vi "Kv_correz_2024.vi"(2 "3rd ac pressure Virial \"G\" (Pa^-2)":dbl, 3 "Pressure [Pa]":dbl, 4 "2nd ac pressure Virial \"F\" (Pa^-1)":dbl) -> (1 "Kv":dbl)   [LabVIEW 2016]
uses:
  2022/SOS_Global_2022.vi
panel:
  out "Kv (ppm)":dbl
  out "3rd vir contr to Kv":dbl
  out "2nd vir contr to kV":dbl format="%#_6e"
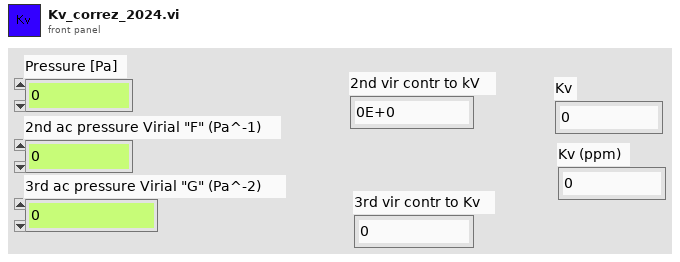
[diagram p1: front panel]
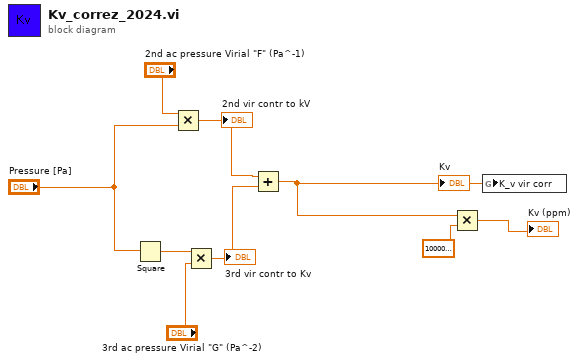
[diagram p0: block diagram]
diagram:
  n1 = Square(x="Pressure [Pa]") -> (x^2=w9:dbl)
  n2 = Multiply(x="2nd ac pressure Virial \"F\" (Pa^-1)", y="Pressure [Pa]") -> (x*y=w7:dbl)
  "2nd vir contr to kV" <- w7
  n3 = Multiply(x=w9, y="3rd ac pressure Virial \"G\" (Pa^-2)") -> (x*y=w6:dbl)
  "3rd vir contr to Kv" <- w6
  n4 = Add(x=w7, y=w6) -> (x+y=w3:dbl)
  "Kv" <- w3
  n5 = Multiply(x=w3, y=1000000.0) -> (x*y=→"Kv (ppm)":dbl)
  n6 = global write "SOS_Global_2022.vi" "K_v vir corr"(w3) -> ()
